vi "DriveArc.vi"(11 "DriveBase.lvclass":refnum<class "DriveBase.lvclass">) -> (3 "DriveBase.lvclass":refnum<class "DriveBase.lvclass">)   [LabVIEW 2016, in "DriveBase.lvclass"]
uses:
  DriveBase.lvclass
panel:
  in  "angleSetpointInput":dbl
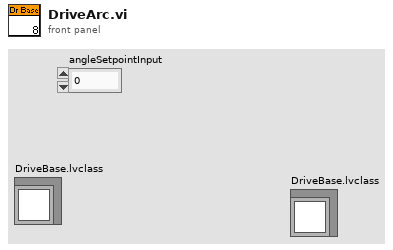
[diagram p1: front panel]
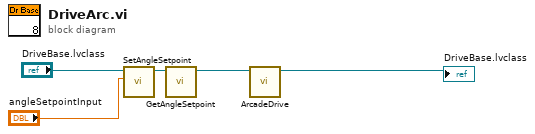
[diagram p0: block diagram]
diagram:
  n1 = call "SetAngleSetpoint.vi"("angleSetpointInput"="angleSetpointInput", "DriveBase.lvclass"="DriveBase.lvclass") -> ("DriveBase.lvclass"=w5:refnum<class "DriveBase.lvclass">)  [unwired: 9 in]
  n2 = call "GetAngleSetpoint.vi"("DriveBase.lvclass"=w5) -> ("DriveBase.lvclass"=w3:refnum<class "DriveBase.lvclass">)  [unwired: 9 in, 1 out]
  n3 = call "ArcadeDrive.vi"("DriveBase.lvclass 2"=w3) -> ("DriveBase.lvclass"=→"DriveBase.lvclass":refnum<class "DriveBase.lvclass">)  [unwired: 10 in]
